vi "Initialize Settings 1.0.vi"(8 "error in (no error)":errorcluster, 11 "settings 1.0":cluster{"key":string, "value":string}[](array[cluster])) -> (0 "error out":errorcluster, 3 "configuration 1.0":T1)   [LabVIEW 2020, in "DSF Core.lvlib" / "Channel Configuration.lvclass"]
uses:
  Channel Configuration.lvclass
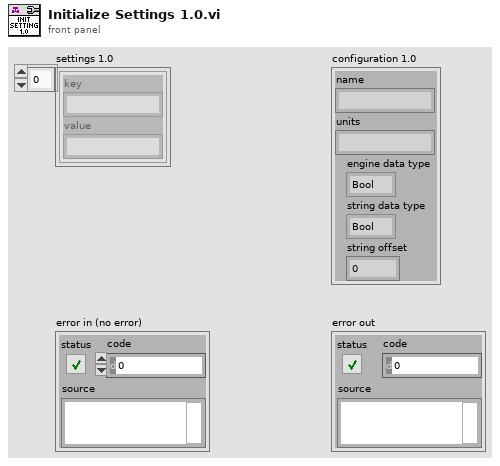
[diagram p1: front panel]
types:
  T1 = cluster{"name":string, "units":string, "engine data type":enum8{"Bool", "SGL", "DBL", "I8", "I16", "I32", "I64", "U8", "U16", "U32", "U64"}, "string data type":enum8{"Bool", "SGL", "DBL", "I8", "I16", "I32", "I64", "U8", "U16", "U32", "U64"}, "string offset":u64}
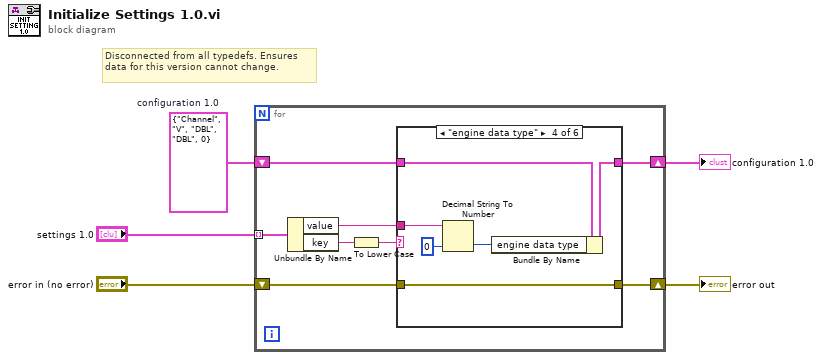
[diagram p0: block diagram]
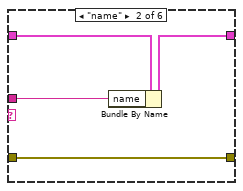
[diagram p3: hidden frame]
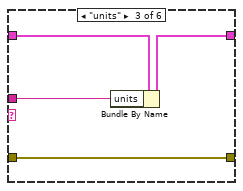
[diagram p4: hidden frame]
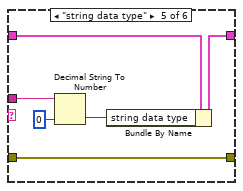
[diagram p5: hidden frame]
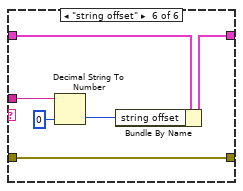
[diagram p6: hidden frame]
diagram:
  w2 = T1 {"name"="Channel", "units"="V", "engine data type"=enum."DBL", "string data type"=enum."DBL", "string offset"=0}  # configuration 1.0
  # "Disconnected from all typedefs. Ensures data for this version cannot change."
  n1 = for {
    shift-right: [w6] -> w5
    shift-left: "error in (no error)" -> [w12]
    shift-right: [w8] -> w3
    shift-left: w2 -> [w9]
    tunnel: "settings 1.0" -> [w13] mode=indexing
    n2 = Unbundle By Name(w13) -> ("value"=w10:string, "key"=w11:string)
    n3 = To Lower Case(string=w11) -> (all lower case string=w7:string)
    n4 = case shown="\"engine data type\"" w7 {
      tunnel: w12 -> [w14 w16 w20 w27 w33 w39]
      tunnel: w10 -> [_ w17 w21 w26 w32 w38]
      tunnel: w9 -> [w15 w19 w23 w29 w35 w41]
      tunnel: [w15 w18 w22 w28 w34 w40] -> w8
      tunnel: [w14 w16 w20 w27 w33 w39] -> w6
      frame Default {
        # "Unknown Setting."
      }
      frame "name" {
        n5 = Bundle By Name(cluster=w19, "name"=w17) -> (w18:T1)
      }
      frame "units" {
        n6 = Bundle By Name(cluster=w23, "units"=w21) -> (w22:T1)
      }
      frame "engine data type" {
        n7 = Decimal String To Number(string=w26, default (0L)=u8 0 ("default (0 I32)")) -> (number=w25:u8)  [unwired: 1 in, 1 out]
        n8 = Bundle By Name(cluster=w29, "engine data type"=w25) -> (w28:T1)
      }
      frame "string data type" {
        n9 = Decimal String To Number(string=w32, default (0L)=u8 0 ("default (0 I32)")) -> (number=w31:u8)  [unwired: 1 in, 1 out]
        n10 = Bundle By Name(cluster=w35, "string data type"=w31) -> (w34:T1)
      }
      frame "string offset" {
        n11 = Decimal String To Number(string=w38, default (0L)=u64 0 ("default (0 I32)")) -> (number=w37:u64)  [unwired: 1 in, 1 out]
        n12 = Bundle By Name(cluster=w41, "string offset"=w37) -> (w40:T1)
      }
    }
  }
  "error out" <- w5
  "configuration 1.0" <- w3
